vi "Set Level.vi"(8 "error in (no error)":errorcluster, 10 "Level":T1(ring), 11 "Record.Error in":refnum<class "Record.Error.lvclass">) -> (0 "error out":errorcluster, 3 "Record.Error out":refnum<class "Record.Error.lvclass">)   [LabVIEW 2017]
uses:
  Record.Error.lvclass
  \\192.168.1.40\Neosoft/Partage/Dossiers Personnels/BRO/DevTools_BR/wc/Error Handler/Record/Record.lvclass
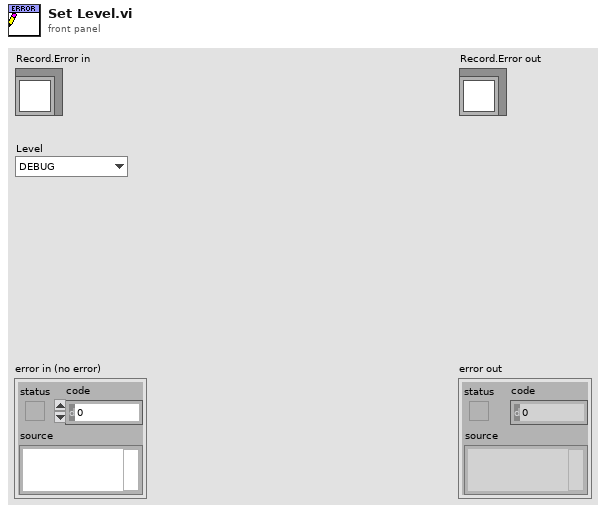
[diagram p1: front panel]
types:
  T1 = enum16{"DEBUG", "INFO", "WARNING", "ERROR", "CRITICAL"}
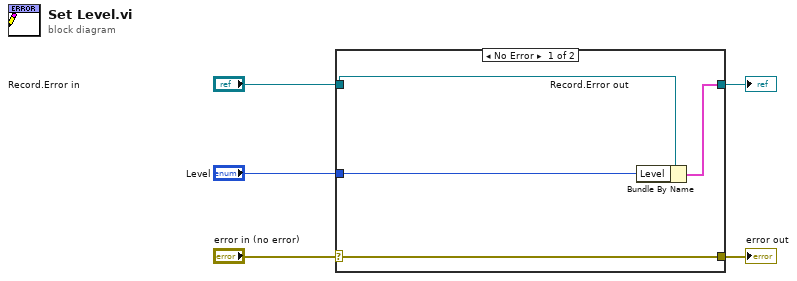
[diagram p0: block diagram]
diagram:
  n1 = case shown="No Error" "error in (no error)" {
    selector: "error in (no error)" -> [w9 w10]
    tunnel: [w9 w10] -> w4
    tunnel: [w7 w11] -> w2
    tunnel: "Record.Error in" -> [w8 w11]
    tunnel: "Level" -> [w6 _]
    frame No Error {
      n2 = Bundle By Name(cluster=w8, "Level"=w6) -> (w7:cluster{})
    }
    frame Error {
    }
  }
  "error out" <- w4
  "Record.Error out" <- w2
